vi "Master_DataStream.vi"(8 "error in":errorcluster, 9 "reader name in":refnum<k21>, 10 "Enum in":T1) -> (0 "error out":errorcluster, 1 "reader name out":refnum<k21>, 2 "Enum out":T1, 3 "Boolean":bool)   [LabVIEW 2018]
doc: "Data streams for cRIO."
uses:
  Host/Libraries/TypeDef_NetworkStreamState.ctl
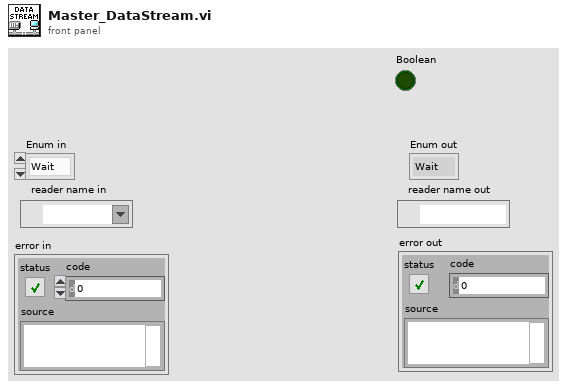
[diagram p1: front panel]
types:
  T1 = typedef "TypeDef_NetworkStreamState.ctl" = enum16{"Wait", "Test", "Initialize", "Read/Write", "Terminate"}
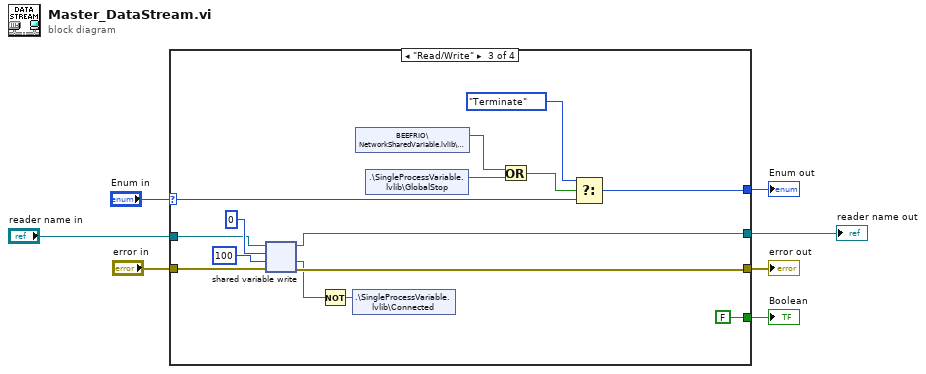
[diagram p0: block diagram]
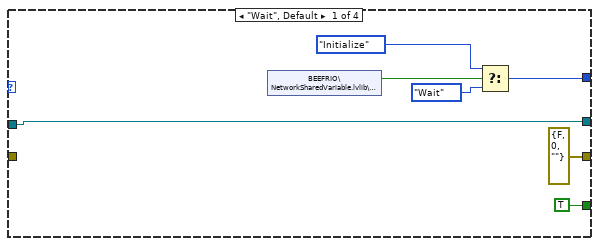
[diagram p2: hidden frame]
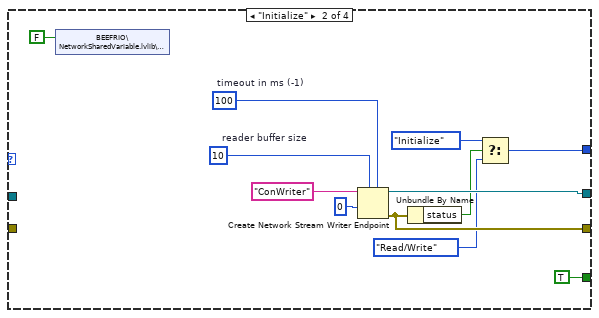
[diagram p3: hidden frame]
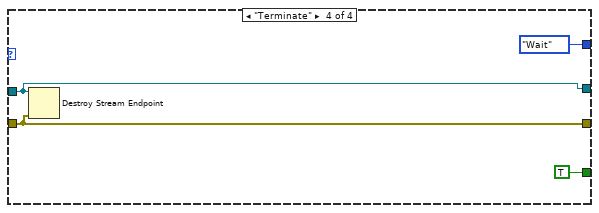
[diagram p4: hidden frame]
diagram:
  n1 = case shown="\"Read/Write\"" "Enum in" {
    selector: "Enum in" -> [_ _ w41 _]
    tunnel: [w14 w26 w31 w45] -> w2
    tunnel: [errorcluster {"status"=FALSE, "code"=0, "source"=""} ("error IO") w25 w32 w43] -> w7
    tunnel: "error in" -> [_ _ w30 w43]
    tunnel: "reader name in" -> [w14 _ w29 w45]
    tunnel: [w10 w21 w39 TypeDef_NetworkStreamState."Wait"] -> w5
    tunnel: [TRUE TRUE FALSE TRUE] -> w1
    frame "Wait", Default {
      n2 = shared-variable "BEEFRIO\\NetworkSharedVariable.lvlib\\ReIntStreams"() -> (w8:bool)  [unwired: 1 in, 1 out]
      n3 = Select(t=TypeDef_NetworkStreamState."Initialize", s=w8, f=TypeDef_NetworkStreamState."Wait") -> (s? t:f=w10:T1)
    }
    frame "Initialize" {
      w17 = 100  # timeout in ms (-1)
      w18 = 10  # reader buffer size
      n4 = shared-variable "BEEFRIO\\NetworkSharedVariable.lvlib\\ReIntStreams"(FALSE ("ReintStreams")) -> ()  [unwired: 1 in, 1 out]
      n5 = Create Network Stream Writer Endpoint(5:w17, 7:w18, 9:i8 0, 11:"ConWriter" ("reader name")) -> (0:w25:errorcluster, 3:w26:refnum<k21>)  [unwired: 3 in]
      n6 = Unbundle By Name(w25) -> ("status"=w24:bool)
      n7 = Select(t=TypeDef_NetworkStreamState."Initialize" ("Enum"), s=w24, f=TypeDef_NetworkStreamState."Read/Write" ("Enum")) -> (s? t:f=w21:T1)
    }
    frame "Read/Write" {
      n8 = shared-variable-write(w29, w30, i8 0, 100 ("timeout ms (-1)")) -> (w31:refnum<k21>, w32:errorcluster, w27:bool)
      n9 = Not(x=w27) -> (.not. x?=w28:bool)
      n10 = shared-variable ".\\SingleProcessVariable.lvlib\\Connected"(w28) -> ()  [unwired: 1 in, 1 out]
      n11 = shared-variable "BEEFRIO\\NetworkSharedVariable.lvlib\\ReIntStreams"() -> (w33:bool)  [unwired: 1 in, 1 out]
      n12 = shared-variable ".\\SingleProcessVariable.lvlib\\GlobalStop"() -> (w37:bool)  [unwired: 1 in, 1 out]
      n13 = Or(x=w33, y=w37) -> (x .or. y?=w38:bool)
      n14 = Select(t=TypeDef_NetworkStreamState."Terminate", s=w38, f=w41) -> (s? t:f=w39:T1)
    }
    frame "Terminate" {
      n15 = Destroy Stream Endpoint(8:w43, 11:w45) -> ()  [unwired: 1 out]
    }
  }
  "error out" <- w7
  "Enum out" <- w5
  "reader name out" <- w2
  "Boolean" <- w1
